vi "Auto_Routine_BlueStraightTwoPieceCenterMoveCenterLineTRAJ.vi"(8 "error in (no error)":errorcluster) -> (0 "error out":errorcluster)   [LabVIEW 2023]
uses:
  Trajectory/TrajectoryGlobals.vi
  <vilib>/Rock Robotics/WPI/ThirdParty/JAS_Junk/TrajLib/Trajectory_Library.lvlib
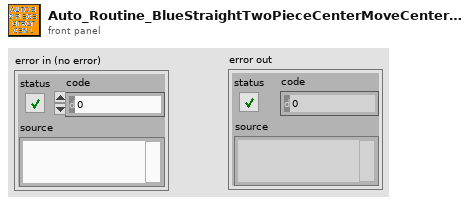
[diagram p1: front panel]
types:
  T1 = typedef "Trajectory_Library.lvlib/TRAJECTORY.ctl" = cluster{"TotalTImeSecs":dbl, "States":T2[]}
  T2 = typedef "Trajectory_Library.lvlib/TRAJ_STATE.ctl" = cluster{"TimeSeconds":dbl, "Velocity":dbl, "Acceleration":dbl, "POSE":T3, "Curvature":dbl}
  T3 = typedef "Trajectory_Library.lvlib/POSE2D.ctl" = cluster{"TRANSLATION":T4, "ROTATION":T5}
  T4 = typedef "Trajectory_Library.lvlib/TRANSLATION2D.ctl" = cluster{"X":dbl, "Y":dbl}
  T5 = typedef "Trajectory_Library.lvlib/ROTATION2D.ctl" = cluster{"VALUE":dbl, "COS":dbl, "SIN":dbl}
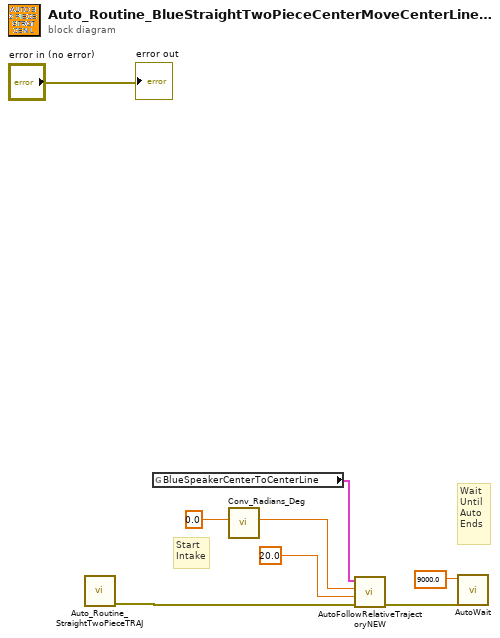
[diagram p0: block diagram]
diagram:
  # "Start\nIntake"
  # "Wait\nUntil\nAuto \nEnds"
  n1 = call "Auto_Routine_StraightTwoPieceTRAJ.vi"() -> ("error out"=w1:errorcluster)  [unwired: 11 in]
  n2 = global read "TrajectoryGlobals.vi" "BlueSpeakerCenterToCenterLine"() -> (w6:T1)
  n3 = call <vilib>:"Conv_Radians_Deg.vi"("Radians"=0.0) -> ("Degrees"=w4:dbl)  [unwired: 10 in]
  n4 = call "AutoFollowRelativeTrajectoryNEW.vi"("error in (no error)"=w1, "TimeOut (s)"=20.0, "End Orientation"=w4, "Trajectory"=w6) -> ("error out"=w2:errorcluster)  [unwired: 7 in]
  n5 = call "AutoWait.vi"("error in (no error)"=w2, "TimeOut (s)"=9000.0) -> ()  [unwired: 9 in, 1 out]
  "error out" <- "error in (no error)"
